vi "Data Logger Loop.vi"   [LabVIEW 2013]
uses:
  Data Logger Mode.ctl
types:
  T1 = typedef "Data Logger Mode.ctl" = enum16{"Init", "Main", "Start", "Stop"}
  T2 = typedef "Pump Data.ctl" = cluster{"Voltages":dbl[], "PumpCurrent":dbl[], "Speed":dbl[], "ControllerCurrent":dbl[], "Pressure":dbl[], "Flow":dbl[], "Elapsed Time (Display)":dbl[], "Avg Pressure":dbl, "Avg Speed":dbl, "Elapsed Time":dbl[]}
  T3 = typedef "Tank Data.ctl" = cluster{"PS Actual (V):":dbl, "Temp1":dbl, "Temp2":dbl}
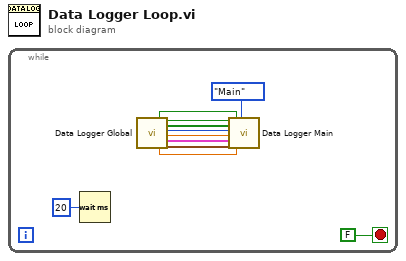
[diagram p0: block diagram]
diagram:
  n1 = while {
    stop <- FALSE stop-if-true
    n2 = Wait (ms)(milliseconds to wait=u32 20) -> ()  [unwired: 1 out]
    n3 = call "Data Logger Global.vi"() -> ("Concat Data OUT"=w1:bool, "Record Time (sec) OUT"=w2:dbl, "WebDAV Push OUT"=w9:bool, "In Spec OUT"=w4:bool[], "Current Step OUT"=w8:i32, "Step Time Left OUT"=w7:dbl, "Pump Data OUT"=w6:T2, "Tank Data OUT"=w5:T3)  [unwired: 12 in]
    n4 = call "Data Logger Main.vi"("WebDAV Push"=w9, "In Spec"=w4, "Current Step"=w8, "Step Time Left"=w7, "Pump Data"=w6, "Tank Data"=w5, "Concat Data"=w1, "Record Time (sec)"=w2, "Data Logger Mode"=Data_Logger_Mode."Main") -> ()  [unwired: 11 in]
  }
